vi "FFT x(t) to dB,Degrees (2D).vi"(8 "Fs (Hz)":dbl=1.0, 11 "X(t)":dbl[][](array[numeric]) format="%.2f") -> (0 "Freq (Hz)":dbl[](array[numeric]), 2 "+Freq Phase of FFT (degrees)":dbl[][](array[numeric]) format="%.2f", 3 "+Freq. Mag of FFT (dB rms)":dbl[][](array[numeric]) format="%.2f")   [LabVIEW 2020]
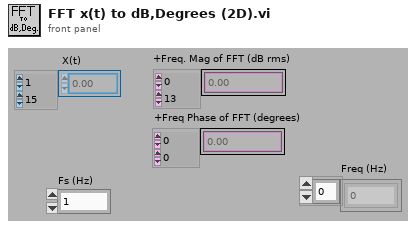
[diagram p1: front panel]
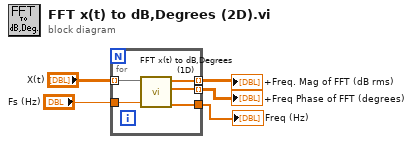
[diagram p0: block diagram]
diagram:
  n1 = for {
    tunnel: "X(t)" -> [w10] mode=indexing
    tunnel: [w9] -> w5 mode=indexing
    tunnel: [w8] -> w4 mode=indexing
    tunnel: "Fs (Hz)" -> [w7]
    tunnel: [w6] -> w1
    n2 = call "FFT x(t) to dB,Degrees (1D).vi"("Fs (Hz)"=w7, "X"=w10) -> ("Freq (Hz)"=w6:dbl[], "+Freq Phase of FFT (degrees)"=w8:dbl[], "+Freq. Mag of FFT (dB rms)"=w9:dbl[])  [unwired: 7 in]
  }
  "+Freq. Mag of FFT (dB rms)" <- w5
  "+Freq Phase of FFT (degrees)" <- w4
  "Freq (Hz)" <- w1
